vi "Save_filename_List.vi"(1 "append to file? (new file:F)":bool=TRUE, 2 "Filename to save":path[](array[path]), 3 "file path (dialog if empty)":path) -> ()   [LabVIEW 2010]
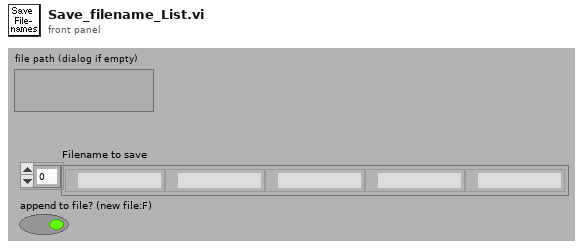
[diagram p1: front panel]
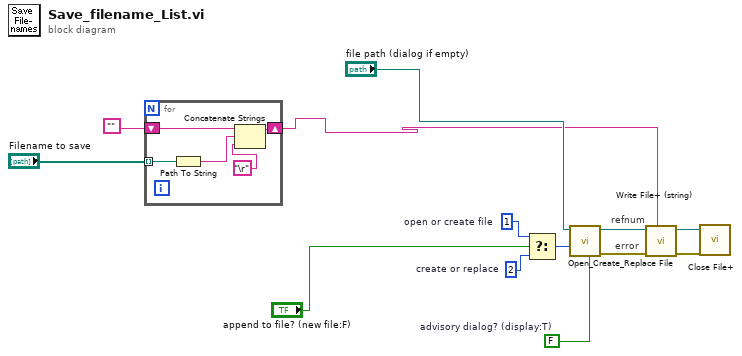
[diagram p0: block diagram]
diagram:
  w3 = FALSE  # advisory dialog? (display:T)
  w10 = i16 2  # create or replace
  w9 = i16 1  # open or create file
  # "error"
  # "refnum"
  n1 = for {
    shift-right: [w15] -> w1
    shift-left: "" -> [w18]
    tunnel: "Filename to save" -> [w14] mode=indexing
    n2 = Path To String(path=w14) -> (string=w17:string)
    n3 = Concatenate Strings(w18, w17, "\r") -> (w15:string)
  }
  n4 = Select(t=w9, s="append to file? (new file:F)", f=w10) -> (s? t:f=w8:i16)
  n5 = call <vilib>:"Open_Create_Replace File.vi"("advisory dialog? (display:T)"=w3, "function (open:0)"=w8, "file path"="file path (dialog if empty)") -> ("error out"=w5:errorcluster, "refnum"=w11:refnum<file>)  [unwired: 4 in, 3 out]
  n6 = call <vilib>:"Write File+ (string).vi"("string"=w1, "error in (no error)"=w5, "refnum"=w11) -> ("error out"=w6:errorcluster, "dup refnum"=w7:refnum<file>)  [unwired: 2 in, 3 out]
  n7 = call <vilib>:"Close File+.vi"("error in (no error)"=w6, "refnum"=w7) -> ()  [unwired: 6 out]
